vi "Apply Label Policy.vi"(9 "String":string, 10 "type descriptor":i16[](array[numeric]), 11 "StringFormatter":refnum<class "StringFormatter.lvclass">) -> (1 "Labeled String":string, 3 "StringFormatter out":refnum<class "StringFormatter.lvclass">)   [LabVIEW 2020, in "OpenStringFormatter.lvlib" / "StringFormatter.lvclass"]
uses:
  StringFormatter.lvclass
  StringFormatter.lvclass/StringFormatter.ctl
  _built_ppls/OpenDescriptor.lvlibp/TypeDescriptor_GetPString.vi
  _built_ppls/OpenDescriptor.lvlibp
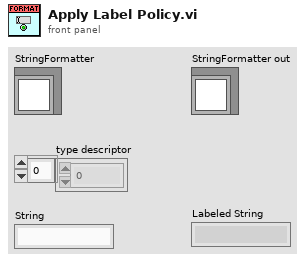
[diagram p1: front panel]
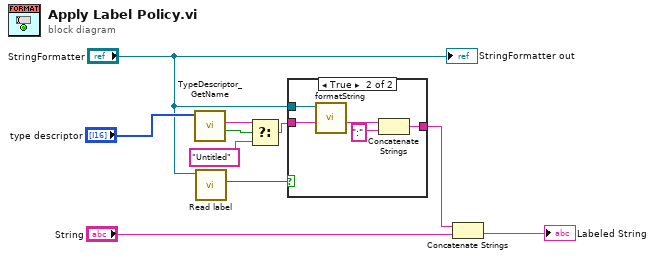
[diagram p0: block diagram]
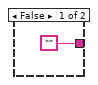
[diagram p2: hidden frame]
diagram:
  n1 = call "TypeDescriptor_GetName.vi"("type descriptor"="type descriptor") -> ("found"=w7:bool, "name"=w8:string)  [unwired: 8 in, 1 out]
  n2 = call "Read label.vi"("StringFormatter in"="StringFormatter") -> ("label"=w2:bool)  [unwired: 9 in, 1 out]
  n3 = Select(t=w8, s=w7, f="Untitled" ("format string")) -> (s? t:f=w9:string)
  n4 = case shown="True" w2 {
    tunnel: ["" w16] -> w4
    tunnel: "StringFormatter" -> [_ w15]
    tunnel: w9 -> [_ w14]
    frame False {
    }
    frame True {
      n5 = call-dynamic "formatString.vi"("Value"=w14, "StringFormatter"=w15) -> ("Formatted Value"=w13:string)  [unwired: 9 in]
      n6 = Concatenate Strings(w13, ":" ("format string")) -> (w16:string)
    }
  }
  n7 = Concatenate Strings(w4, "String") -> (→"Labeled String":string)
  "StringFormatter out" <- "StringFormatter"
